vi "multicolumn.vi"() -> ()   [LabVIEW 2018]
panel:
  out "x+1":i32
  out "array":i32[](array[numeric])
  out "Numeric 3":i32
  out "Numeric 2":i32
  out "lm35 2":i32
  in  "Multicolumn Listbox":i32(listbox)
  out "appended array":string[][](array[string])
  in  "pt100":dbl[](array[numeric])
  in  "ntc":dbl[](array[numeric])
  in  "lm35":dbl[](array[numeric])
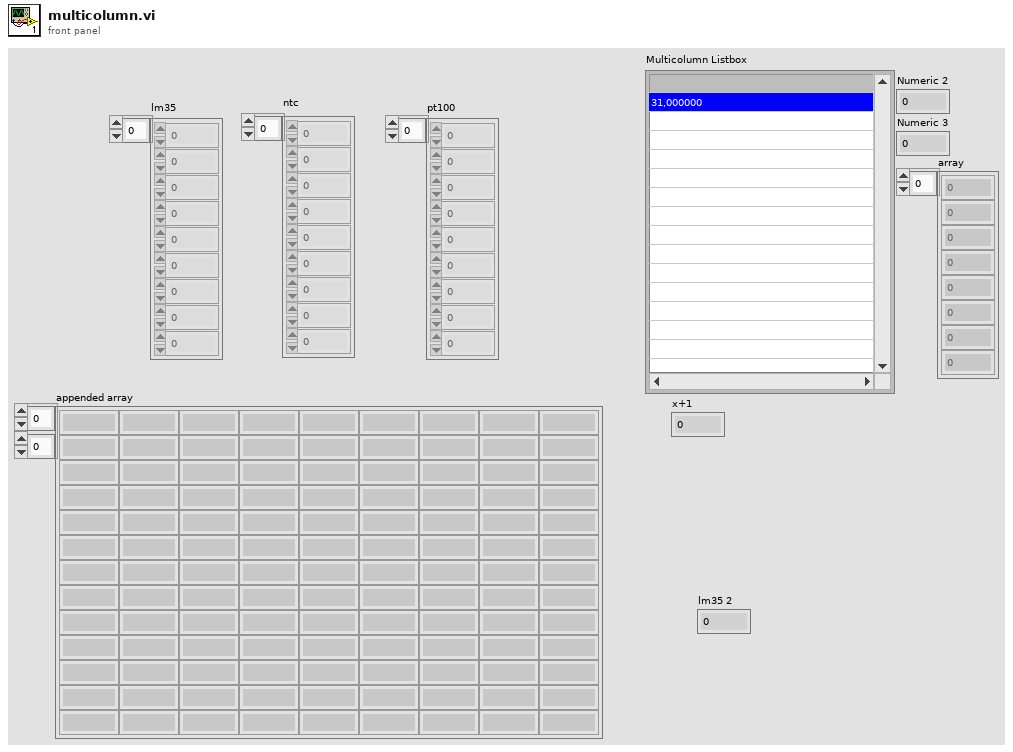
[diagram p1: front panel]
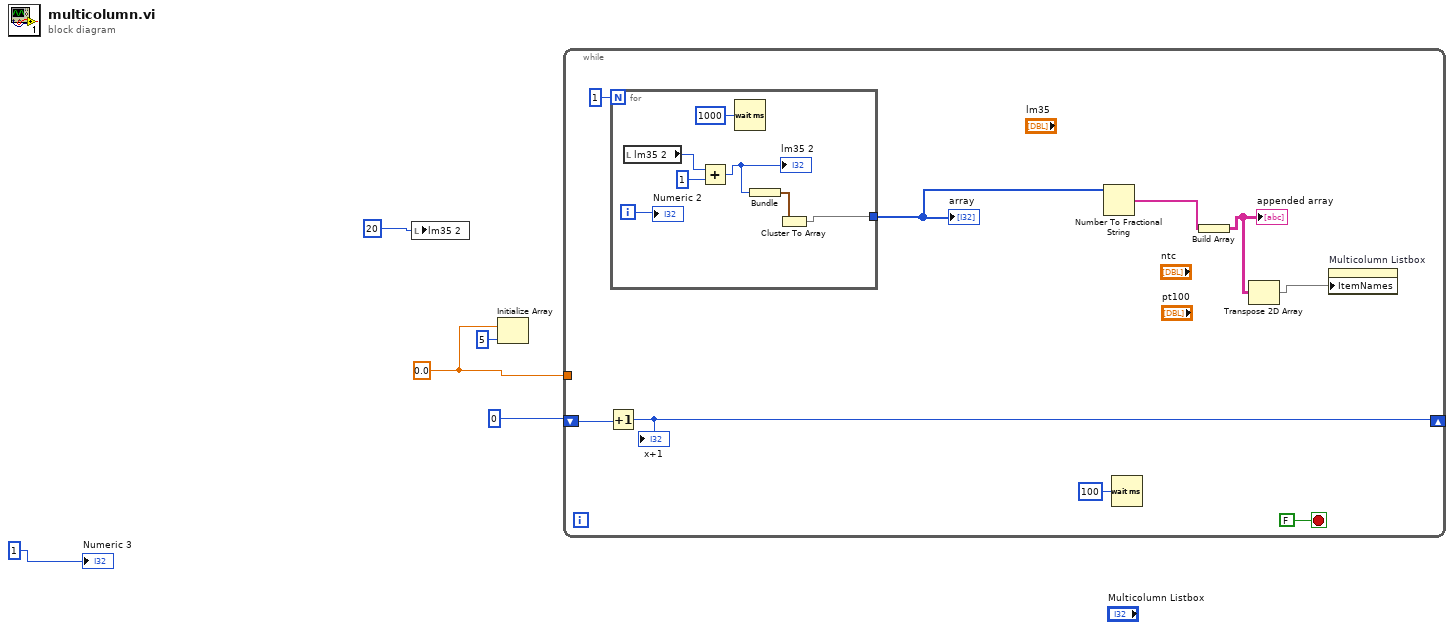
[diagram p0: block diagram]
diagram:
  w2 = 0.0 ("element")
  n1 = local write "lm35 2"(20 ("lm35 2")) -> ()
  n2 = Initialize Array(w2, 5 ("dimension size")) -> ()  [unwired: 1 out]
  n3 = while {
    shift-right: [w9] -> _
    shift-left: 0 ("lm35 2") -> [w10]
    tunnel: w2 -> [_]
    stop <- FALSE stop-if-true
    n4 = Increment(x=w10) -> (x+1=w9:i32)
    "x+1" <- w9
    n5 = for {
      N: 1 -> [_]
      tunnel: [w15] -> w8
      i -> [w18]
      n6 = local read "lm35 2"() -> (w19:i32)
      n7 = Add(x=w19, y=1) -> (x+y=w17:i32)
      "lm35 2" <- w17
      n8 = Wait (ms)(milliseconds to wait=u32 1000) -> ()  [unwired: 1 out]
      n9 = Bundle(w17) -> (w16:cluster{i32})  [unwired: 1 in]
      n10 = Cluster To Array(cluster=w16) -> (array=w15:i32[])
      "Numeric 2" <- w18
    }
    "array" <- w8
    n11 = Number To Fractional String(number=w8) -> (F-format string=w13:string[])  [unwired: 3 in]
    n12 = Wait (ms)(milliseconds to wait=u32 100) -> ()  [unwired: 1 out]
    n13 = Build Array(w13) -> (w7:string[][])
    "appended array" <- w7
    n14 = Transpose 2D Array(2D array=w7) -> (transposed array=w6:string[][])
    n15 = property on="Multicolumn Listbox" class="MCListbox (strict)"("ItemNames"=w6) -> ()  [unwired: 2 in, 2 out]
  }
  "Numeric 3" <- 1 ("Numeric 3")
